vi "Humidity Max Read.vi"   [LabVIEW 2023, in "Climate Chamber.lvclass"]
uses:
  Climate Chamber.lvclass
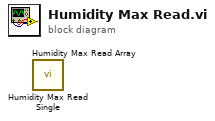
[diagram p0: block diagram]
diagram:
  n1 = call "Humidity Max Read Single.vi"() -> ()  [unwired: 8 in, 4 out]
  n2 = call "Humidity Max Read Array.vi"() -> ()  [unwired: 8 in, 4 out]
